vi "Date_jours.vi"(6 "year":i32, 7 "fractional second":dbl, 8 "jours n":i32, 9 "hour":i32, 10 "minute":i32, 11 "second":i32) -> (3 "horodatage":timestamp)   [LabVIEW 2015]
uses:
  <vilib>/Utility/miscctls.llb/LVDateTimeRec.ctl
panel:
  in  "cluster date/heure":T1
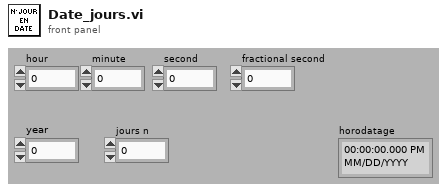
[diagram p1: front panel]
types:
  T1 = typedef "LVDateTimeRec.ctl" = cluster{"fractional second":dbl, "second":i32, "minute":i32, "hour":i32, "day of month":i32, "month":i32, "year":i32, "day of week":i32, "day of year":i32, "DST":i32}
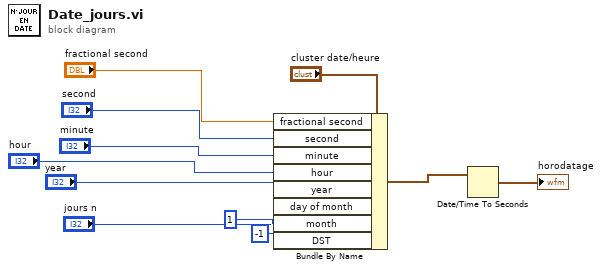
[diagram p0: block diagram]
diagram:
  n1 = Bundle By Name(cluster="cluster date/heure", "fractional second"="fractional second", "second"="second", "minute"="minute", "hour"="hour", "year"="year", "day of month"="jours n", "month"=1, "DST"=-1) -> (w10:T1)
  n2 = Date/Time To Seconds(2:w10) -> (0:→"horodatage":timestamp)  [unwired: 1 out]
